vi "FP midbrain THINK.vi"(2 "GPS  Initial":cluster{"X pos":i32, "Y pos":i32, "Heading":dbl}, 5 "Tried Docking?":bool, 6 "error in":errorcluster, 7 "GPS":cluster{"X pos":i32, "Y pos":i32, "Heading":dbl}, 8 "Forebrain Comd":T2, 9 "IR Sensors":T3(array[cluster]), 10 "Camera Data":T1) -> (0 "error out":errorcluster, 1 "Behavior\nVelocity OUT":dbl, 3 "Behavior arrays":T4, 4 "Don't Use Forebrain ACT?":bool)   [LabVIEW 2014]
doc: "This vi is the midbrain THINK routine. It selects the behaviors which the boat will use based upon the passed Forebrain Command."
panel:
  in  "Radius":dbl=60.0 format="%#_13g"
  out "Waveform Graph":cluster{dbl, dbl, dbl[][]}(graph)
  # "(Current)"
  # "(Dock)"
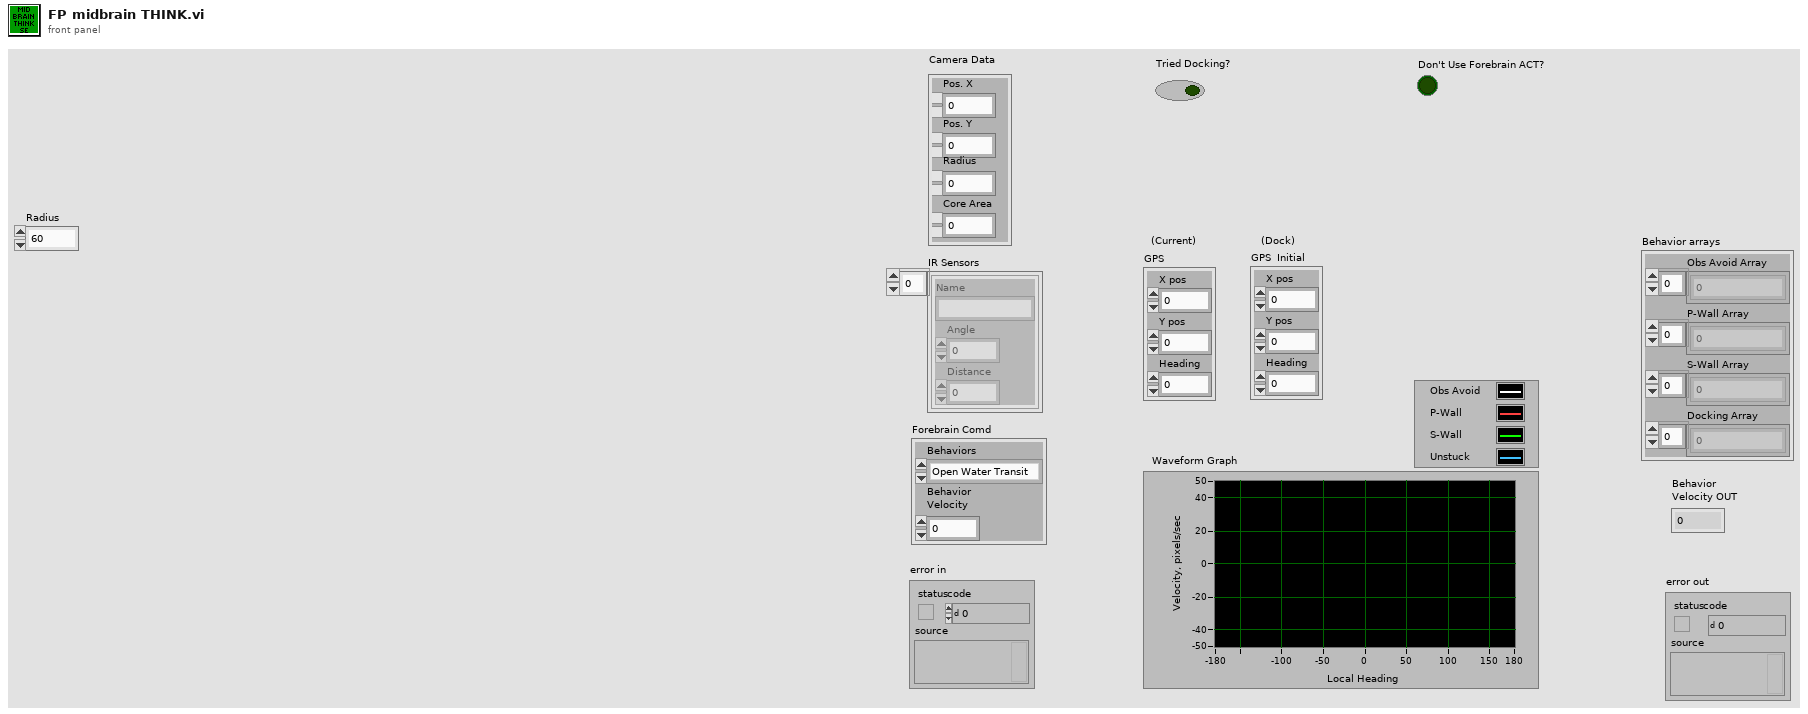
[diagram p1: front panel]
types:
  T1 = cluster{"Pos. X":i32, "Pos. Y":i32, "Radius":i32, "Core Area":i32}
  T2 = cluster{"Behaviors":enum16{"Open Water Transit", "P-Wall Follow", "S-Wall Follow", "Dock", "Chase"}, "Behavior\nVelocity":dbl}
  T3 = cluster{"Name":string, "Angle":dbl, "Distance":dbl}[]
  T4 = cluster{"Obs Avoid Array":dbl[], "P-Wall Array":dbl[], "S-Wall Array":dbl[], "Docking Array":dbl[]}
  T5 = enum16{"Open Water Transit", "P-Wall Follow", "S-Wall Follow", "Dock", "Chase"}
  T6 = cluster{"Obstacle Avoidance":bool, "P-Wall Follow":bool, "S-Wall Follow":bool, "Point to Dock":bool}
  T7 = cluster{"Obs Avoid Array":dbl[], "P-Wall Array":dbl[], "S-Wall Array":dbl[], "Dock Array":dbl[]}
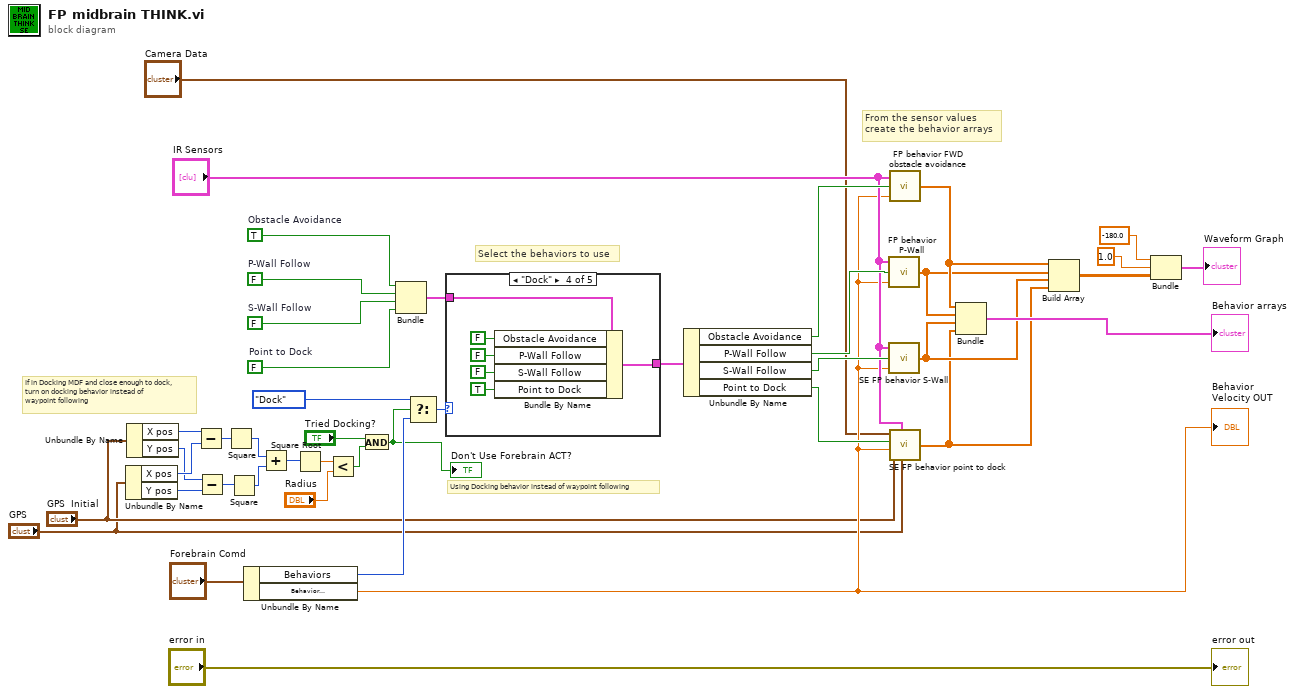
[diagram p0: block diagram]
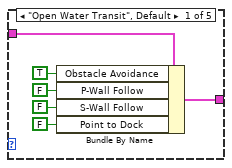
[diagram p2: hidden frame]
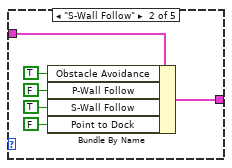
[diagram p3: hidden frame]
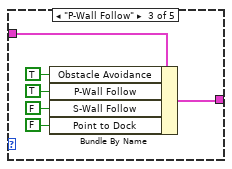
[diagram p4: hidden frame]
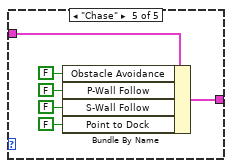
[diagram p5: hidden frame]
diagram:
  w39 = FALSE  # Point to Dock
  w40 = FALSE  # S-Wall Follow
  w41 = FALSE  # P-Wall Follow
  w42 = TRUE  # Obstacle Avoidance
  # "Using Docking behavior instead of waypoint following"
  # "If in Docking MDF and close enough to dock,\nturn on docking behavior instead of \nwaypoint following"
  # "From the sensor values\ncreate the behavior arrays"
  # "Select the behaviors to use"
  n1 = Unbundle By Name("GPS") -> ("X pos"=w7:i32, "Y pos"=w5:i32)
  n2 = Unbundle By Name("GPS  Initial") -> ("X pos"=w8:i32, "Y pos"=w6:i32)
  n3 = Subtract(x=w8, y=w7) -> (x-y=w17:i32)
  n4 = Subtract(x=w6, y=w5) -> (x-y=w16:i32)
  n5 = Square(x=w17) -> (x^2=w15:i32)
  n6 = Square(x=w16) -> (x^2=w14:i32)
  n7 = Unbundle By Name("Forebrain Comd") -> ("Behaviors"=w21:T5, "Behavior\nVelocity"=w22:dbl)
  "Behavior\nVelocity OUT" <- w22
  n8 = Add(x=w15, y=w14) -> (x+y=w11:i32)
  n9 = Square Root(x=w11) -> (sqrt(x)=w13:dbl)
  n10 = Less?(x=w13, y="Radius") -> (x < y?=w3:bool)
  n11 = And(x="Tried Docking?", y=w3) -> (x .and. y?=w2:bool)
  "Don't Use Forebrain ACT?" <- w2
  n12 = Bundle("Obstacle Avoidance"=w42, "P-Wall Follow"=w41, "S-Wall Follow"=w40, "Point to Dock"=w39) -> (w38:T6)  [unwired: 1 in]
  n13 = Select(t=T5."Dock" ("Behaviors"), s=w2, f=w21) -> (s? t:f=w19:T5)
  n14 = case shown="\"Dock\"" w19 {
    tunnel: w38 -> [w49 w55 w61 w67 w69]
    tunnel: [w47 w53 w59 w65 w68] -> w1
    frame "Open Water Transit", Default {
      n15 = Bundle By Name(cluster=w49, "Obstacle Avoidance"=TRUE, "P-Wall Follow"=FALSE, "S-Wall Follow"=FALSE, "Point to Dock"=FALSE ("Get Unstuck")) -> (w47:T6)
    }
    frame "S-Wall Follow" {
      n16 = Bundle By Name(cluster=w55, "Obstacle Avoidance"=TRUE, "P-Wall Follow"=FALSE, "S-Wall Follow"=TRUE, "Point to Dock"=FALSE ("Get Unstuck")) -> (w53:T6)
    }
    frame "P-Wall Follow" {
      n17 = Bundle By Name(cluster=w61, "Obstacle Avoidance"=TRUE, "P-Wall Follow"=TRUE, "S-Wall Follow"=FALSE, "Point to Dock"=FALSE ("Get Unstuck")) -> (w59:T6)
    }
    frame "Dock" {
      n18 = Bundle By Name(cluster=w67, "Obstacle Avoidance"=FALSE, "P-Wall Follow"=FALSE, "S-Wall Follow"=FALSE, "Point to Dock"=TRUE ("Get Unstuck")) -> (w65:T6)
    }
    frame "Chase" {
      n19 = Bundle By Name(cluster=w69, "Obstacle Avoidance"=FALSE, "P-Wall Follow"=FALSE, "S-Wall Follow"=FALSE, "Point to Dock"=FALSE ("Get Unstuck")) -> (w68:T6)
    }
  }
  n20 = Unbundle By Name(w1) -> ("Obstacle Avoidance"=w37:bool, "P-Wall Follow"=w35:bool, "S-Wall Follow"=w36:bool, "Point to Dock"=w23:bool)
  n21 = call "FP behavior P-Wall.vi"("Behavior\nVelocity"=w22, "Activate?"=w35, "IR Sensors"="IR Sensors") -> ("P-Wall Array"=w29:dbl[])
  n22 = call "SE FP behavior S-Wall.vi"("Behavior\nVelocity"=w22, "Activate?"=w36, "IR Sensors"="IR Sensors") -> ("S-Wall Array"=w27:dbl[])
  n23 = call "FP behavior FWD obstacle avoidance.vi"("Behavior\nVelocity"=w22, "Activate?"=w37, "IR Sensors"="IR Sensors") -> ("Obs Avoid Array"=w30:dbl[])
  n24 = call "SE FP behavior point to dock.vi"("GPS"="GPS", "IR Sensors"="IR Sensors", "GPS Initial"="GPS  Initial", "Behavior\nVelocity"=w22, "Activate?"=w23, "Camera Data"="Camera Data") -> ("Dock Array"=w26:dbl[])
  n25 = Bundle("Obs Avoid Array"=w30, "P-Wall Array"=w29, "S-Wall Array"=w27, "Dock Array"=w26) -> (→"Behavior arrays":T7)  [unwired: 1 in]
  n26 = Build Array(w30, w29, w27, w26) -> (w28:dbl[][])
  n27 = Bundle(-180.0, 1.0, w28) -> (→"Waveform Graph":cluster{dbl, dbl, dbl[][]})  [unwired: 1 in]
  "error out" <- "error in"
